vi "Receive DAC Command.vi"(10 "Consumer Queues in":T1) -> (0 "error out":errorcluster, 2 "Consumer Queues out":T1, 3 "DAC Process Command out":refnum<class "Generic DAC Process Command.lvclass">)   [LabVIEW 2019, in "DAC Process.lvlib" / "Generic DAC Process Command.lvclass"]
uses:
  Generic DAC Process Command.lvclass
  TS Framework/Consumer Queues.ctl
  UI Process/Generic UI Command/Generic UI Process Command.lvclass
  Trig Process/Generic Trig Command/Generic Trig Process Command.lvclass
  TS Framework/TS Framework.lvlib
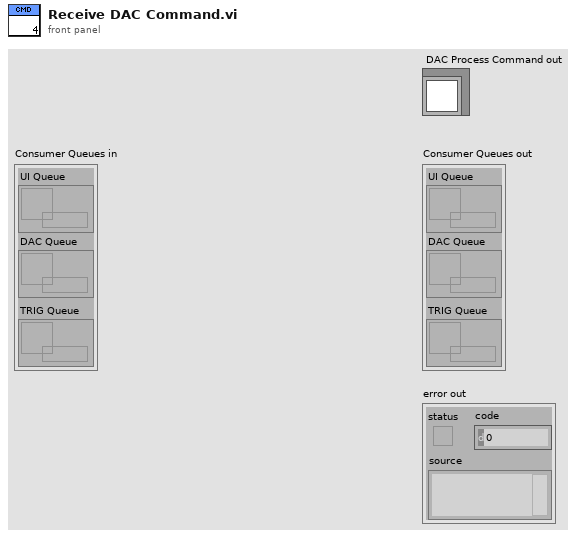
[diagram p1: front panel]
types:
  T1 = typedef "TS Framework.lvlib/Consumer Queues.ctl" = cluster{"UI Queue":refnum<queue>, "DAC Queue":refnum<queue>, "TRIG Queue":refnum<queue>}
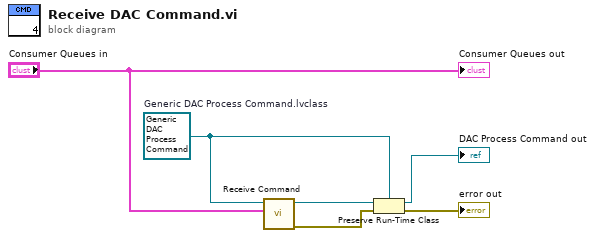
[diagram p0: block diagram]
diagram:
  w1 = refnum<class "Generic DAC Process Command.lvclass"> refnum  # Generic DAC Process Command.lvclass
  n1 = call-dynamic "Receive Command.vi"("Consumer Queues"="Consumer Queues in", "DAC Process Command in"=w1) -> ("error out"=w5:errorcluster, "Generic Command out"=w4:refnum<class "Generic Command.lvclass">)  [unwired: 8 in]
  n2 = Preserve Run-Time Class(object in=w4, error in=w5, 2:w1) -> (object out=→"DAC Process Command out":refnum<class "Generic DAC Process Command.lvclass">, error out=→"error out":errorcluster)
  "Consumer Queues out" <- "Consumer Queues in"
